vi "test-mergeVAttributes.vi"() -> ()   [LabVIEW 2019, in "lv-apt-json-file-test.lvlib"]
uses:
  lv-apt-json-file-test.lvlib
  lv-apt-json-file.lvlib
panel:
  out "data":variant
  out "AttrMap A after B->A":variant
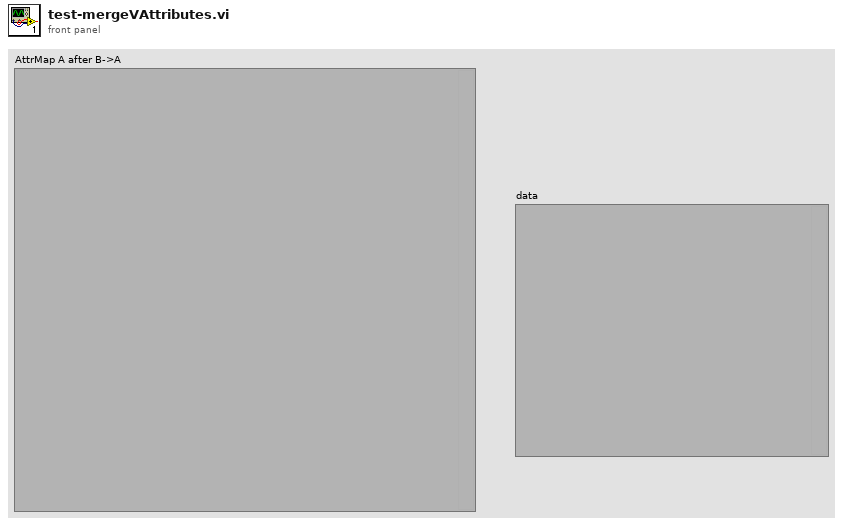
[diagram p1: front panel]
types:
  T1 = cluster{"bool":bool, "string":string, "cluster":cluster{"numeric":i32, "string":string, "cluster":cluster{"numeric":i32, "string":string, "cluster":cluster{"numeric":i32, "string":string}}}}
  T2 = cluster{"numeric":i32, "string":string, "cluster":cluster{"numeric":i32, "string":string, "cluster":cluster{"numeric":i32, "string":string, "cluster":cluster{"numeric":i32, "string":string}}}}
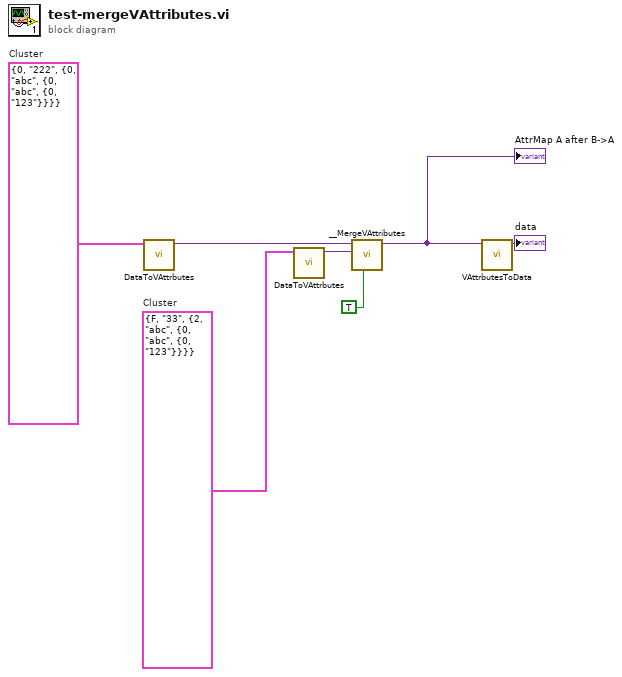
[diagram p0: block diagram]
diagram:
  w6 = T1 {"bool"=FALSE, "string"="33", "cluster"={"numeric"=2, "string"="abc", "cluster"={"numeric"=0, "string"="abc", "cluster"={"numeric"=0, "string"="123"}}}}  # Cluster
  w7 = T2 {"numeric"=0, "string"="222", "cluster"={"numeric"=0, "string"="abc", "cluster"={"numeric"=0, "string"="abc", "cluster"={"numeric"=0, "string"="123"}}}}  # Cluster
  n1 = call "DataToVAttrbutes.vi"("data"=w7) -> ("VAttributes"=w4:variant)  [unwired: 9 in, 1 out]
  n2 = call "DataToVAttrbutes.vi"("data"=w6) -> ("VAttributes"=w5:variant)  [unwired: 9 in, 1 out]
  n3 = call "__MergeVAttributes.vi"("If exist? Skip(T)/Overwrite(F)"=TRUE, "VAttributes B"=w5, "VAttributes A"=w4) -> ("VAttributes A after B->A"=w3:variant)  [unwired: 7 in, 1 out]
  "AttrMap A after B->A" <- w3
  n4 = call "VAttrbutesToData.vi"("VAttributes"=w3) -> ("data"=→"data":variant)  [unwired: 9 in, 1 out]
